vi "ShooterSpeedDebugV4.1.vi"(8 "Reset PID":bool) -> (2 "Wheel 1 Actual Voltage":dbl=11.112915570970326, 3 "GO GO GO":bool=TRUE)   [LabVIEW 2012]
uses:
  Robot Global Data.vi
  Max'sToolKit/ConvertPercentVbusToVoltage.vi
  Max'sToolKit/ConvertVoltageToPercentVbs.vi
panel:
  out "Spin Up Time (s)":dbl=0.32156799999984287
  out "Loop Rate (Hz)":dbl=99.14634998450656
  in  "Filter Size":i8=1
  in  "Wheel 1 Out-->PID":dbl=0.2 format="%.2f"
  in  "Wheel 1 Index":i8
  in  "Wheel 1 PID-->Out":dbl=10.0 format="%.2f"
  in  "Use PID":bool=TRUE
  out "Motor Outputs":cluster{"Error":dbl, dbl, "x":dbl}(graph)={"Error"=0.01927161419290968, 33.338746712910975, "x"=0.0}
  in  "Tolerence (+/-) RPS":dbl=0.5
  out "Wheel 1 Error":dbl=0.01927161419290968
  in  "Wheel 1 Setpoint":dbl format="%.2f"
  in  "W1 PID gains":T1={"proportional gain (Kc)"=0.07, "integral time (Ti, min)"=0.0, "derivative time (Td, min)"=0.050000000000000024} {"derivative time (Td, min)" format="%.6f"; "integral time (Ti, min)" format="%.6f"; "proportional gain (Kc)" format="%.6f"}
  in  "Wheel 1 Feed Foward":dbl format="%_6g"
  out "Wheel 1 Output":dbl=0.9328122435011209
  out "Wheel 1 RPM":dbl=61.98072838580709
  # "spin up time includes 1/4 sec\nmakesure good delay"
  # "66.5 RPS for close 3pt between 7.4 and 6.65 volts"
  # "32.5 RPS --> ~7.1 volts filter of 1\n62.0 RPS --> ~11.5 volts filter 1-ish gets noisy"
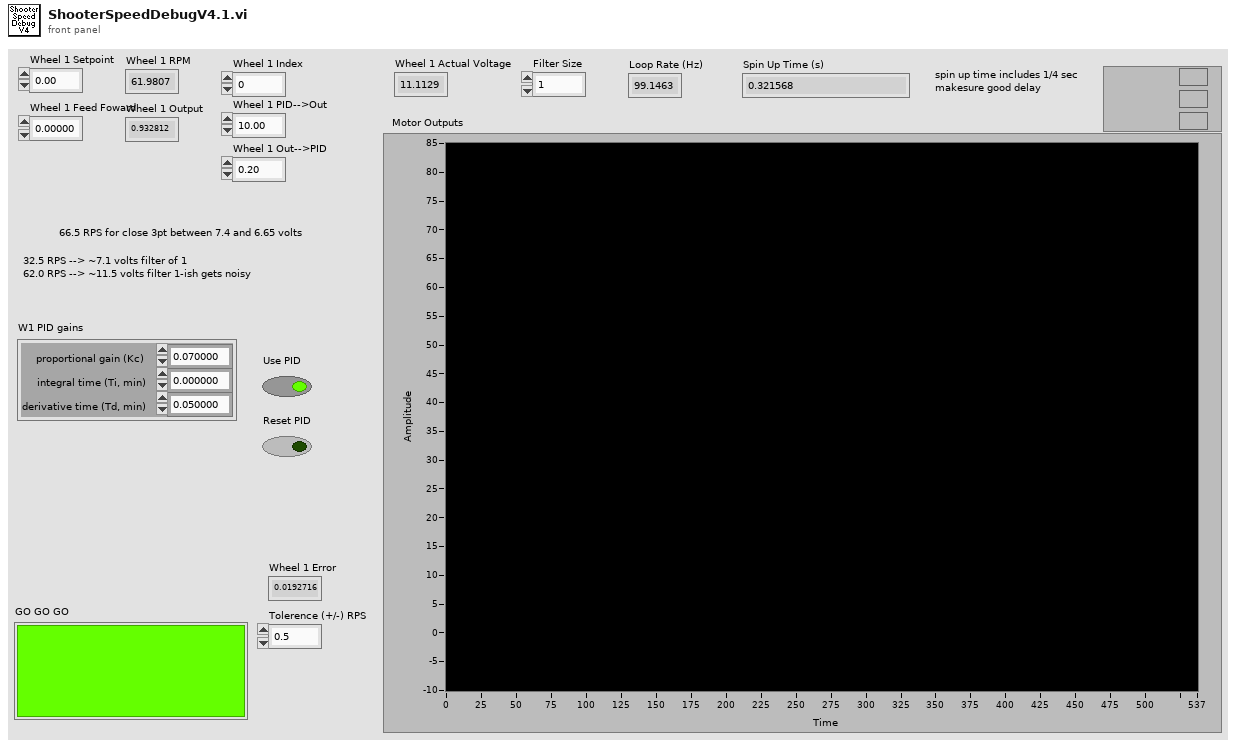
[diagram p1: front panel]
types:
  T1 = cluster{"proportional gain (Kc)":dbl, "integral time (Ti, min)":dbl, "derivative time (Td, min)":dbl}
  T2 = typedef "WPI_EncoderDevRef.ctl" = cluster{"DevStatus":errorcluster, "EncoderIndex":T3, "CounterIndex":T4, "DistancePerCount":dbl, "Decoding Type":T5}
  T3 = typedef "FPGA_EncoderIdx.ctl" = enum8{"Enc 0", "Enc 1", "Enc 2", "Enc 3", "Invalid"}
  T4 = typedef "FPGA_CounterCtrSystemIndex.ctl" = enum8{"Ctr 0", "Ctr 1", "Ctr 2", "Ctr 3", "Ctr 4", "Ctr 5", "Ctr 6", "Ctr 7", "Invalid"}
  T5 = typedef "WPI_EncoderType.ctl" = enum16{"1x", "2x", "4x"}
  T6 = cluster{"Wheel 1 PID-->Out":dbl, "Wheel 1 Out-->PID":dbl}
  T7 = typedef "WPI_MotorControlDeviceRef.ctl" = cluster{"DeviceStatus":errorcluster, "Type":enum16{"PWM", "CAN"}, "PWM":cluster{"Digital Module":T8, "PWM Channel":T9, "DeadBand":T10}, "CAN":cluster{"Device Number":u8, "Control Mode":T11, "Semaphore":T12, "Max Vout":dbl}, "Invert":bool, "TransformRef":T13, "InvTransformRef":T13}
  T8 = typedef "FPGA_TypedefDigitalModule.ctl" = enum16{"Digital Module 1", "Digital Module 2"}
  T9 = typedef "FPGA_DIOPWMChannel.ctl" = enum8{"PWM 1", "PWM 2", "PWM 3", "PWM 4", "PWM 5", "PWM 6", "PWM 7", "PWM 8", "PWM 9", "PWM 10", "Invalid"}
  T10 = typedef "WPI_PWMDeadband.ctl" = cluster{"Name":string, "maxPositivePwm":i32, "minPositivePwm":i32, "centerPwm":i32, "maxNegativePwm":i32, "minNegativePwm":i32, "angularRange":u16}
  T11 = typedef "WPI_CANJaguar_ControlMode.ctl" = enum8{"Percent VBus", "Current", "Speed", "Position", "Voltage"}
  T12 = typedef "Semaphore RefNum" = refnum<k1>
  T13 = typedef "WPI_PWMTransform_ConPane.ctl" = refnum<vi>
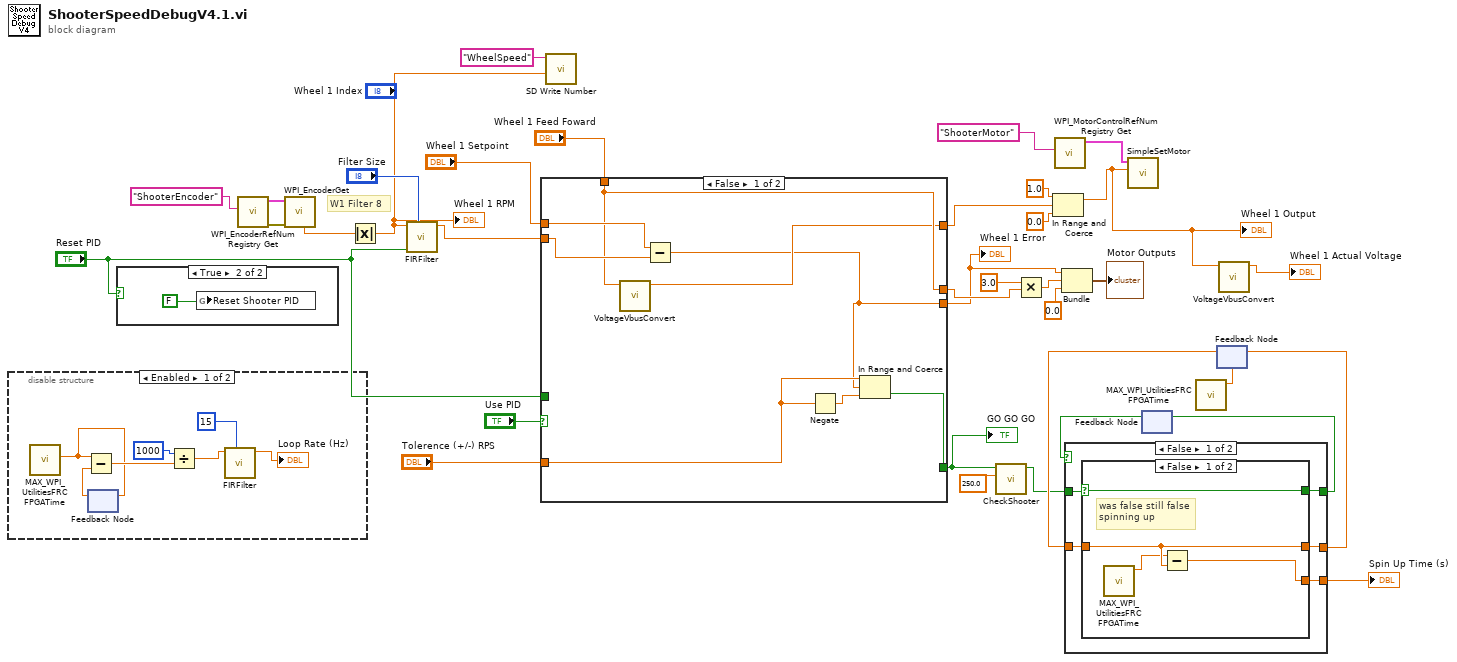
[diagram p0: block diagram]
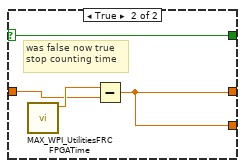
[diagram p2: hidden frame]
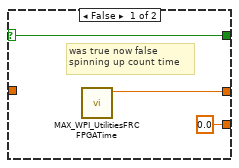
[diagram p4: hidden frame]
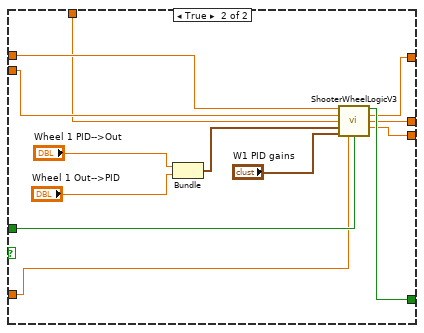
[diagram p7: hidden frame]
diagram:
  # "W1 Filter 8"
  n1 = disable-structure shown="Enabled" {
    frame Enabled {
      n2 = call "MAX_WPI_UtilitiesFRC FPGATime.vi"() -> ("FPGA Time (ms)"=w36:dbl)  [unwired: 9 in, 2 out]
      n3 = feedback #1() -> (w40:dbl)  [unwired: 1 in]
      n4 = Subtract(x=w36, y=w40) -> (x-y=w42:dbl)
      n5 = feedback-in #1(w36) -> ()
      n6 = Divide(x=1000, y=w42) -> (x/y=w37:dbl)
      n7 = call "FIRFilter.vi"("Filter Size"=i8 15, "Input"=w37) -> ("Output"=→"Loop Rate (Hz)":dbl)  [unwired: 9 in]
    }
    frame Disabled {
    }
  }
  n8 = case shown="True" "Reset PID" {
    frame False {
    }
    frame True {
      n9 = global write "Robot Global Data.vi" "Reset Shooter PID"(FALSE) -> ()
    }
  }
  n10 = call <vilib>:"WPI_EncoderRefNum Registry Get.vi"("refnum name"="ShooterEncoder") -> ("error out"=w32:errorcluster, "EncoderDevRef"=w33:T2)  [unwired: 9 in]
  n11 = call <vilib>:"WPI_EncoderGet.vi"("error in (no error)"=w32, "EncoderDevRef"=w33) -> ("Rate"=w31:dbl)  [unwired: 4 in, 5 out]
  n12 = Absolute Value(x=w31) -> (abs(x)=w1:dbl)
  "Wheel 1 RPM" <- w1
  n13 = call "FIRFilter.vi"("Filter Size"="Filter Size", "Reset"="Reset PID", "Input"=w1) -> ("Output"=w30:dbl)  [unwired: 8 in]
  n14 = case shown="False" "Use PID" {
    tunnel: [w47 w64] -> w3
    tunnel: w30 -> [w51 w63]
    tunnel: "Tolerence (+/-) RPS" -> [w45 w59]
    tunnel: "Reset PID" -> [_ w60]
    tunnel: "Wheel 1 Setpoint" -> [w50 w62]
    tunnel: "Wheel 1 Feed Foward" -> [w49 w55]
    tunnel: [w48 w54] -> w14
    tunnel: [w49 w53] -> w18
    tunnel: [w44 w52] -> w17
    frame False {
      n15 = call-poly "VoltageVbusConvert.vi"("Voltage"=w49) -> ("Vbus"=w48:dbl)  [unwired: 10 in]
      n16 = Subtract(x=w50, y=w51) -> (x-y=w44:dbl)
      n17 = Negate(x=w45) -> (-x=w46:dbl)
      n18 = In Range and Coerce(upper limit=w45, x=w44, lower limit=w46) -> (In Range?=w47:bool)  [unwired: 1 out]
    }
    frame True {
      n19 = Bundle("Wheel 1 PID-->Out"="Wheel 1 PID-->Out", "Wheel 1 Out-->PID"="Wheel 1 Out-->PID") -> (w56:T6)  [unwired: 1 in]
      n20 = call "ShooterWheelLogicV3.vi"("Setpoint"=w62, "Process Varaible"=w63, "Feedfoward Voltage"=w55, "SwitchZones"=w56, "PID gains"="W1 PID gains", "Error Margin"=w59, "Reset"=w60) -> ("At Speed"=w64:bool, "Motor Output"=w54:dbl, "Voltage Output"=w53:dbl, "Error"=w52:dbl)  [unwired: 4 in, 1 out]
    }
  }
  "Wheel 1 Error" <- w17
  "GO GO GO" <- w3
  n21 = call <vilib>:"SD Write Number.vi"("Numeric"=w1, "Name"="WheelSpeed") -> ()  [unwired: 8 in, 2 out]
  n22 = call "CheckShooter.vi"("Time for happy (ms)"=250.0, "Shooter Good?"=w3) -> ("Good to shoot"=w5:bool)  [unwired: 9 in]
  n23 = Multiply(x=3.0, y=w18) -> (x*y=w22:dbl)
  n24 = In Range and Coerce(upper limit=1.0, x=w14, lower limit=0.0) -> (coerced(x)=w13:dbl)  [unwired: 1 out]
  "Wheel 1 Output" <- w13
  n25 = call <vilib>:"WPI_MotorControlRefNum Registry Get.vi"("refnum name"="ShooterMotor") -> ("MotorControlDevRef"=w27:T7)  [unwired: 9 in, 1 out]
  n26 = Bundle("Error"=w17, w22, "x"=0.0) -> (→"Motor Outputs":cluster{"Error":dbl, dbl, "x":dbl})  [unwired: 1 in]
  n27 = call "SimpleSetMotor.vi"("Output"=w13, "MotorControlDevRef"=w27) -> ()  [unwired: 8 in, 2 out]
  n28 = feedback #2() -> (w11:bool)  [unwired: 1 in]
  n29 = call "MAX_WPI_UtilitiesFRC FPGATime.vi"() -> ("FPGA Time (s)"=w6:dbl)  [unwired: 9 in, 2 out]
  n30 = feedback #3(w6) -> (w8:dbl)
  n31 = case shown="False" w11 {
    tunnel: w5 -> [w69 w82]
    tunnel: [w68 w81] -> w10
    tunnel: [w66 w80] -> w9
    tunnel: w8 -> [w67 w79]
    tunnel: [w65 w78] -> w7
    frame False {
      n32 = case shown="False" w69 {
        selector: w69 -> [w73 w77]
        tunnel: [w73 w77] -> w68
        tunnel: w67 -> [w72 w75]
        tunnel: [w72 w74] -> w66
        tunnel: [w71 w74] -> w65
        frame False {
          # "was false still false\nspinning up"
          n33 = call "MAX_WPI_UtilitiesFRC FPGATime.vi"() -> ("FPGA Time (s)"=w70:dbl)  [unwired: 9 in, 2 out]
          n34 = Subtract(x=w70, y=w72) -> (x-y=w71:dbl)
        }
        frame True {
          # "was false now true\nstop counting time"
          n35 = call "MAX_WPI_UtilitiesFRC FPGATime.vi"() -> ("FPGA Time (s)"=w76:dbl)  [unwired: 9 in, 2 out]
          n36 = Subtract(x=w76, y=w75) -> (x-y=w74:dbl)
        }
      }
    }
    frame True {
      n37 = case shown="True" w82 {
        selector: w82 -> [w85 w87]
        tunnel: [w85 w87] -> w81
        tunnel: [w84 w86] -> w80
        tunnel: w79 -> [_ w86]
        tunnel: [0.0 ("FPGA Time (s)") w86] -> w78
        frame False {
          # "was true now false\nspinning up count time"
          n38 = call "MAX_WPI_UtilitiesFRC FPGATime.vi"() -> ("FPGA Time (s)"=w84:dbl)  [unwired: 9 in, 2 out]
        }
        frame True {
          # "was true still true\nhas spun up"
        }
      }
    }
  }
  "Spin Up Time (s)" <- w7
  n39 = feedback-in #2(w10) -> ()
  n40 = feedback-in #3(w9) -> ()
  n41 = call-poly "VoltageVbusConvert.vi"("Vbus"=w13) -> ("Voltage"=→"Wheel 1 Actual Voltage":dbl)  [unwired: 10 in]
